vi "New Output.vi"(8 "error in (no error)":errorcluster, 11 "Descriptor":string) -> (0 "error out":errorcluster, 3 "output":refnum<class "Output.lvclass">)   [LabVIEW 2015, in "Output.lvclass"]
uses:
  Output.lvclass
  request/request.lvclass
  output_poller/output_poller_queue/output_poller_queue.lvclass
  output_poller/output_poller_queue/output_poller_queue.lvclass/output_poller_queue.ctl
  Output.lvclass/Output.ctl
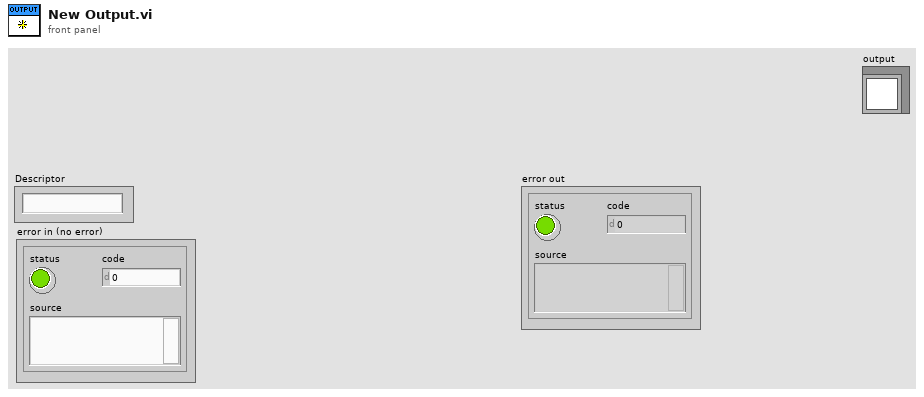
[diagram p1: front panel]
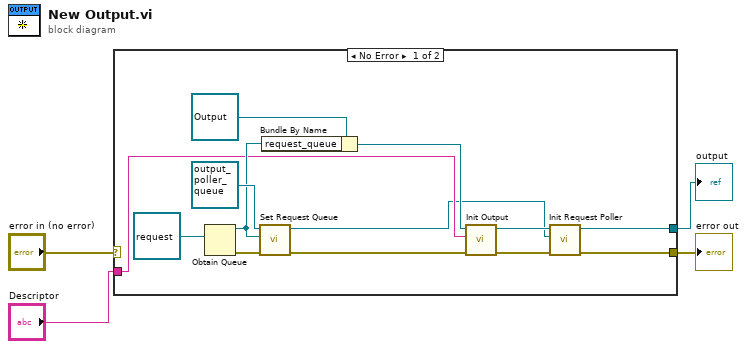
[diagram p0: block diagram]
diagram:
  n1 = case shown="No Error" "error in (no error)" {
    selector: "error in (no error)" -> [_ w18]
    tunnel: "Descriptor" -> [w11 _]
    tunnel: [w6 w18] -> w3
    tunnel: [w5 _] -> w1
    frame No Error {
      n2 = Obtain Queue(element data type=refnum<class "request.lvclass"> refnum ("request.lvclass")) -> (queue out=w12:refnum<queue>, error out=w13:errorcluster)  [unwired: 4 in, 1 out]
      n3 = call "Set Request Queue.vi"("error in (no error)"=w13, "request_queue"=w12, "output_poller_queue in"=refnum<class "output_poller_queue.lvclass"> refnum) -> ("error out"=w10:errorcluster, "output_poller_queue out"=w7:refnum<class "output_poller_queue.lvclass">)  [unwired: 7 in]
      n4 = Bundle By Name(cluster=refnum<class "Output.lvclass"> refnum ("output.lvclass"), "request_queue"=w12) -> (w16:refnum<class "Output.lvclass">)
      n5 = call "Init Output.vi"("error in (no error)"=w10, "Descriptor"=w11, "output in"=w16) -> ("error out"=w8:errorcluster, "output out"=w9:refnum<class "Output.lvclass">)  [unwired: 7 in]
      n6 = call "Init Request Poller.vi"("error in (no error)"=w8, "output_request_poller in"=w7, "output in"=w9) -> ("error out"=w6:errorcluster, "output out"=w5:refnum<class "Output.lvclass">)  [unwired: 7 in]
    }
    frame Error {
    }
  }
  "error out" <- w3
  "output" <- w1
